vi "Write data value reference.vi"(8 "error in (no error)":errorcluster, 10 "data value reference":refnum<data-value>, 11 "command_parser in":refnum<class "command_parser.lvclass">) -> (0 "error out":errorcluster, 3 "command_parser out":refnum<class "command_parser.lvclass">)   [LabVIEW 2025, in "command_parser.lvlib" / "command_parser.lvclass"]
uses:
  command_parser.lvclass
  command_parser.lvclass/command_parser.ctl
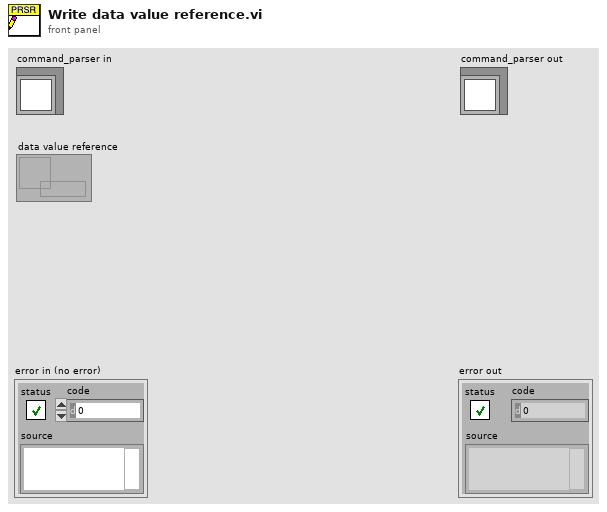
[diagram p1: front panel]
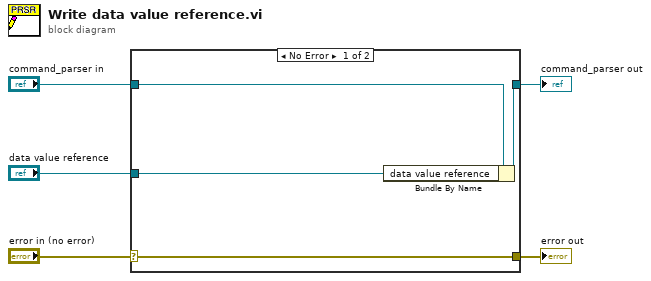
[diagram p0: block diagram]
diagram:
  n1 = case shown="No Error" "error in (no error)" {
    selector: "error in (no error)" -> [w9 w10]
    tunnel: [w9 w10] -> w4
    tunnel: [w7 w11] -> w2
    tunnel: "command_parser in" -> [w8 w11]
    tunnel: "data value reference" -> [w6 _]
    frame No Error {
      n2 = Bundle By Name(cluster=w8, "data value reference"=w6) -> (w7:refnum<class "command_parser.lvclass">)
    }
    frame Error {
    }
  }
  "error out" <- w4
  "command_parser out" <- w2
